vi "Test.vi"() -> ()   [LabVIEW 2017]
uses:
  project/Utilities/Create Linear Vector by Samples.vi
  project/Subsystems/Measurement.PhotocurrentMapping.UI/Measurement.PhotocurrentMapping.UI.lvclass
panel:
  out "LIA ColorBar":T1(plugin-control) caption="SMU ColorBar"
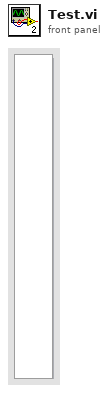
[diagram p1: front panel]
types:
  T1 = typedef "IMAQ Image.ctl" = refnum<image>
  T2 = typedef "Image Type" = u32
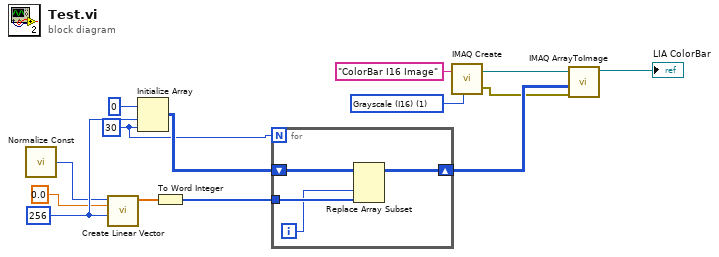
[diagram p0: block diagram]
diagram:
  w6 = T2 1 items=["Grayscale (U8)", "Grayscale (I16)", "Grayscale (SGL)", "Complex (CSG)", "RGB (U32)", "HSL (U32)", "RGB (U64)"] ("Image Type")
  w1 = 30 ("dimension size")
  w13 = 256 ("Samples")
  n1 = call "Normalize Const.vi"() -> ("Const"=w8:i32)  [unwired: 1 in]
  n2 = call-poly "Create Linear Vector.vi"("Samples"=w13, "Stop"=0.0 ("Start"), "Start"=w8) -> ("Vector"=w11:dbl[])  [unwired: 6 in, 2 out]
  n3 = Initialize Array "Initialize Array"(i16 0, w13, w1) -> (w12:i16[][])
  n4 = To Word Integer(number=w11) -> (16bit integer=w10:i16[])
  n5 = for {
    N: w1 -> [_]
    tunnel: w10 -> [w17]
    shift-right: [w16] -> w4
    shift-left: w12 -> [w18]
    i -> [w15]
    n6 = Replace Array Subset(array=w18, new element=w17, index (col)=w15) -> (w16:i16[][])  [unwired: 1 in]
  }
  n7 = call "IMAQ Create"("Image Name"="ColorBar I16 Image", "Image Type"=w6) -> ("New Image"=w5:T1, "error out"=w3:errorcluster)  [unwired: 3 in]
  n8 = call "IMAQ ArrayToImage"("error in (no error)"=w3, "Image Pixels (I16)"=w4, "Image"=w5) -> ("Image Out"=→"LIA ColorBar":T1)  [unwired: 7 in, 1 out]
